vi "I2C_0208.vi"() -> ()   [LabVIEW 2021]
doc: "This example demonstrates how to generate a user-defined voltage using the analog output of a DAQ device."
uses:
  <vilib>/Utility/error.llb/DialogType.ctl
  <vilib>/DAQmx/write.llb/DAQmx Write (Digital 1D U32 1Chan NSamp).vi
  <vilib>/DAQmx/create/channels.llb/DAQmx Create Channel (DO-Digital Output).vi
  <vilib>/DAQmx/configure/timing.llb/DAQmx Timing (Sample Clock).vi
  <vilib>/DAQmx/miscellaneous.llb/DAQmx Fill In Error Info.vi
  <vilib>/Utility/file.llb/Read Delimited Spreadsheet (I64).vi
  <vilib>/DAQmx/write.llb/DAQmx Write (Digital 1D U32 NChan 1Samp).vi
  <resource>/objmgr/daqmx.rc
panel:
  out "Time Pass Outside":u32
  out "Time Pass Inside":u32
  in  "lines":tag
  in  "source":tag
  in  "rate":dbl=1000.0 format="%0.2f"
  out "SampClk.Rate":dbl
  out "DUT":i32
  out "Boolean array":bool[](array[boolean])
  in  "STOP":bool
  out "DIO":cluster{i16, i16}(graph)
  in  "file path (dialog if empty)":path=path "C:/Users/Wayne Shih/Downloads/nPM6100 Positron/HTOL/Labview/AWG by USB6259/test.txt"
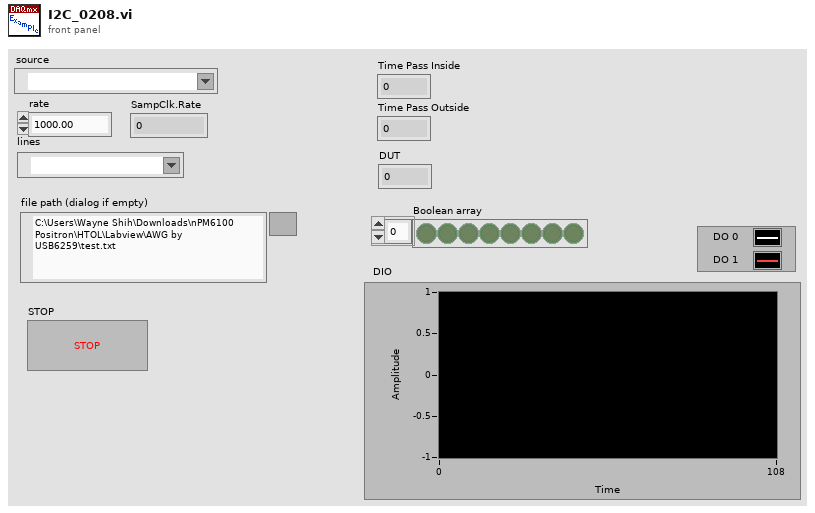
[diagram p1: front panel]
types:
  T1 = typedef "DialogType.ctl" = u16
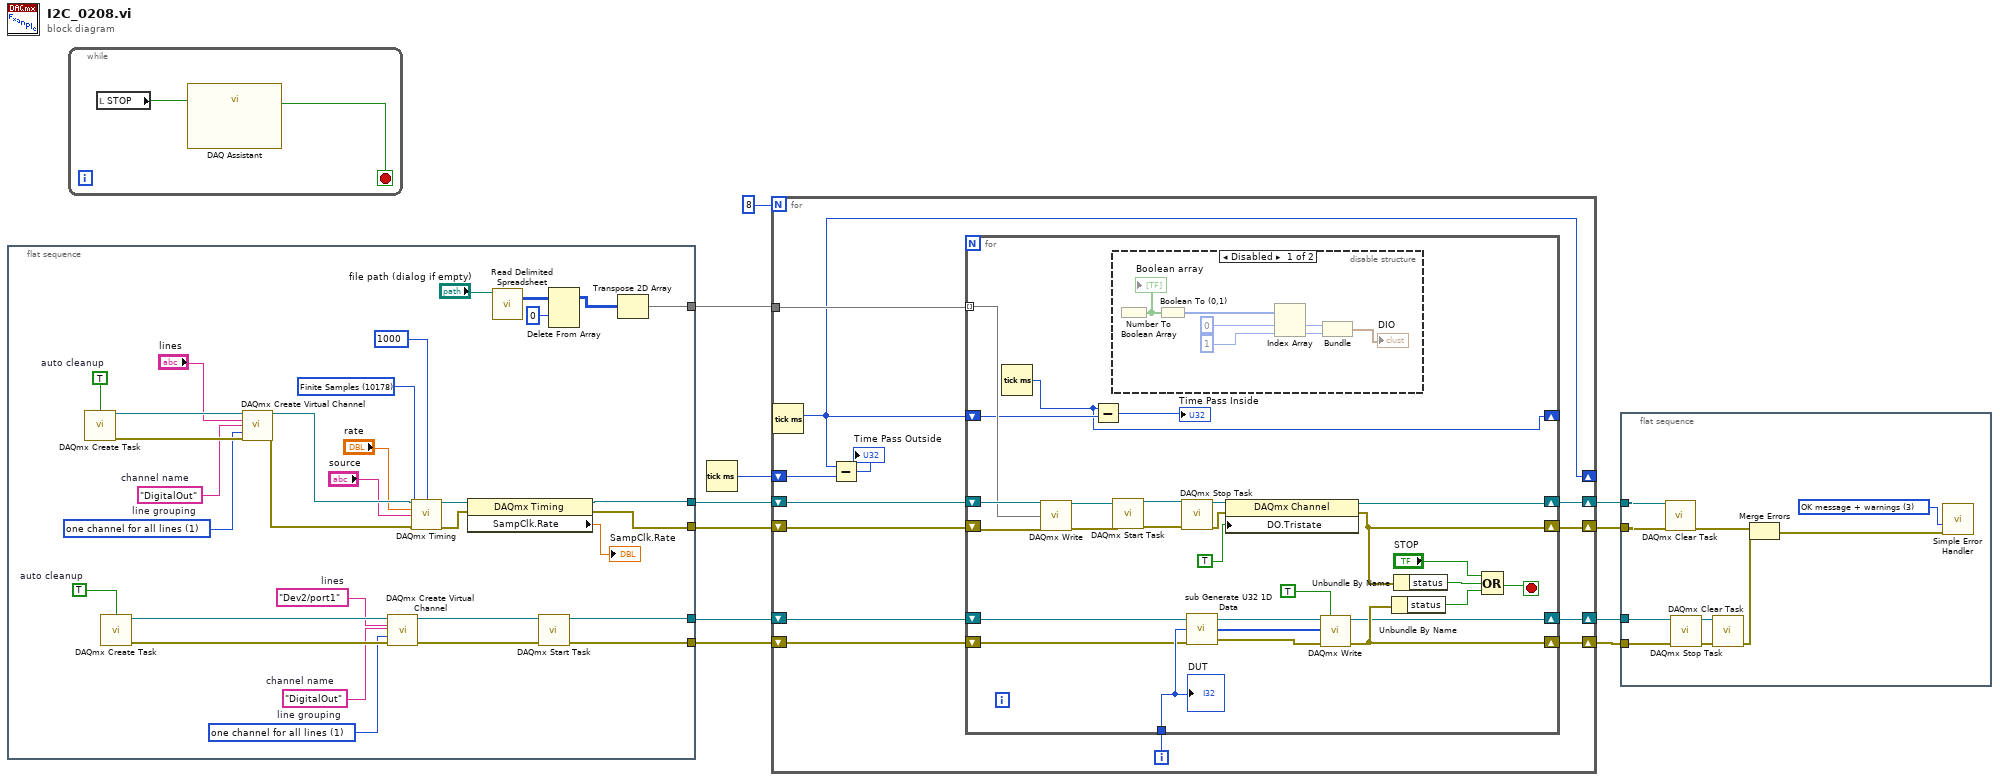
[diagram p0: block diagram]
diagram:
  n1 = flat-sequence {
    tunnel: [w32] -> w11
    tunnel: [w31] -> w10
    tunnel: [w38] -> w8
    tunnel: [w37] -> w7
    tunnel: [w22] -> w2
    frame #0 {
      w15 = 1 items=["one channel for each line", "one channel for all lines"]  # line grouping
      w14 = "DigitalOut"  # channel name
      w16 = "Dev2/port1"  # lines
      w18 = TRUE  # auto cleanup
      w28 = 10178 items=["Finite Samples"=10178, "Continuous Samples"=10123, "Hardware Timed Single Point"=12522] ("sample mode")
      w40 = 1 items=["one channel for each line", "one channel for all lines"]  # line grouping
      w39 = "DigitalOut"  # channel name
      w42 = TRUE  # auto cleanup
      n2 = call <vilib>:"DAQmx Create Task.vi"("auto cleanup"=w42) -> ("task out"=w41:refnum<k21>, "error out"=w43:errorcluster)  [unwired: 13 in]
      n3 = call <vilib>:"DAQmx Create Task.vi"("auto cleanup"=w18) -> ("task out"=w17:refnum<k21>, "error out"=w19:errorcluster)  [unwired: 13 in]
      n4 = call-poly <vilib>:"DAQmx Create Virtual Channel.vi"("task in"=w41, "lines"="lines", "name to assign"=w39, "line grouping"=w40, "error in"=w43) -> ("task out"=w36:refnum<k21>, "error out"=w35:errorcluster)  [unwired: 9 in]
      n5 = call-poly <vilib>:"DAQmx Create Virtual Channel.vi"("task in"=w17, "lines"=w16, "name to assign"=w14, "line grouping"=w15, "error in"=w19) -> ("task out"=w12:refnum<k21>, "error out"=w13:errorcluster)  [unwired: 9 in]
      n6 = call-poly <vilib>:"DAQmx Timing.vi"("task/channels in"=w36, "sample mode"=w28, "samples per channel"=1000, "rate"="rate", "source"="source", "error in"=w35) -> ("task out"=w34:refnum<k21>, "error out"=w33:errorcluster)  [unwired: 8 in]
      n7 = property class="DAQmx Timing"(reference=w34, error in=w33) -> (reference out=w32:refnum<k21>, error out=w31:errorcluster, "SampClk.Rate"=→"SampClk.Rate":dbl)
      n8 = call-poly <vilib>:"Read Delimited Spreadsheet.vi"("file path (dialog if empty)"="file path (dialog if empty)") -> ("all rows"=w25:i64[][])  [unwired: 9 in, 5 out]
      n9 = call <vilib>:"DAQmx Start Task.vi"("task/channels in"=w12, "error in"=w13) -> ("task out"=w38:refnum<k21>, "error out"=w37:errorcluster)  [unwired: 12 in]
      n10 = Delete From Array(array=w25, index (row)=0) -> (array with subset deleted=w24:i64[][])  [unwired: 2 in, 1 out]
      n11 = Transpose 2D Array(2D array=w24) -> (transposed array=w22:i64[][])
    }
  }
  n12 = while {
    stop <- w45 stop-if-true
    n13 = local read "STOP"() -> (w44:bool)
    n14 = call "DAQ Assistant"("stop (F)"=w44) -> ("stopped"=w45:bool)  [unwired: 16 in, 2 out]
  }
  n15 = Tick Count (ms)() -> (millisecond timer value=w1:u32)
  n16 = for {
    N: 8 -> [_]
    shift-right: [w56] -> w4
    shift-left: w11 -> [w58]
    shift-right: [w55] -> w3
    shift-left: w10 -> [w57]
    shift-right: [w51] -> w5
    shift-left: w8 -> [w50]
    shift-right: [w52] -> w6
    shift-left: w7 -> [w53]
    tunnel: w2 -> [w49]
    shift-right: [w47] -> _
    shift-left: w1 -> [w48]
    i -> [w54]
    n17 = Tick Count (ms)() -> (millisecond timer value=w47:u32)
    n18 = Subtract(x=w47, y=w48) -> (x-y=→"Time Pass Outside":u32)
    n19 = for {
      tunnel: w49 -> [w70] mode=indexing
      shift-right: [w60] -> w56
      shift-left: w58 -> [w73]
      shift-right: [w59] -> w55
      shift-left: w57 -> [w72]
      tunnel: w54 -> [w85]
      shift-right: [w82] -> w51
      shift-left: w50 -> [w81]
      shift-right: [w83] -> w52
      shift-left: w53 -> [w84]
      shift-right: [w66] -> _
      shift-left: w47 -> [w68]
      stop <- w71 stop-if-true
      n20 = Tick Count (ms)() -> (millisecond timer value=w66:u32)
      n21 = call-poly <vilib>:"DAQmx Write.vi"("task/channels in"=w73, "data"=w70, "error in"=w72) -> ("task out"=w86:refnum<k21>, "error out"=w69:errorcluster)  [unwired: 10 in, 1 out]
      n22 = Subtract(x=w66, y=w68) -> (x-y=→"Time Pass Inside":u32)
      n23 = disable-structure shown="Disabled" {
        frame Disabled {
          n24 = Number To Boolean Array() -> (Boolean array=w87:bool[])  [unwired: 1 in]
          "Boolean array" <- w87
          n25 = Boolean To (0,1)(Boolean=w87) -> (0, 1=w93:i16[])
          n26 = Index Array(array=w93, index #1=0 ("index"), index #2=1 ("index")) -> (element #1=w90:i16, element #2=w89:i16)
          n27 = Bundle(w90, w89) -> (→"DIO":cluster{i16, i16})  [unwired: 1 in]
        }
        frame Enabled {
        }
      }
      n28 = call <vilib>:"DAQmx Start Task.vi"("task/channels in"=w86, "error in"=w69) -> ("task out"=w64:refnum<k21>, "error out"=w63:errorcluster)  [unwired: 12 in]
      n29 = call <vilib>:"DAQmx Stop Task.vi"("task/channels in"=w64, "error in"=w63) -> ("task out"=w62:refnum<k21>, "error out"=w61:errorcluster)  [unwired: 12 in]
      n30 = call <vilib>:"sub Generate U32 1D Data.vi"("error in"=w84, "initial value"=w85, "task in"=w81) -> ("error out"=w78:errorcluster, "Data"=w77:u32[], "task out"=w76:refnum<k21>)
      n31 = property class="DAQmx Channel"(reference=w62, error in=w61, "DO.Tristate"=TRUE) -> (reference out=w60:refnum<k21>, error out=w59:errorcluster)
      n32 = call-poly <vilib>:"DAQmx Write.vi"("task/channels in"=w76, "auto start"=TRUE, "data"=w77, "error in"=w78) -> ("task out"=w82:refnum<k21>, "error out"=w83:errorcluster)  [unwired: 9 in, 1 out]
      n33 = Unbundle By Name(w83) -> ("status"=w75:bool)
      n34 = Unbundle By Name(w59) -> ("status"=w79:bool)
      n35 = Compound Arithmetic op=OR("STOP", w79, w75) -> (w71:bool)
      "DUT" <- w85
    }
  }
  n36 = flat-sequence {
    tunnel: w4 -> [w95]
    tunnel: w3 -> [w96]
    tunnel: w6 -> [w100]
    tunnel: w5 -> [w99]
    frame #0 {
      w103 = T1 3 items=["no dialog", "OK message", "continue or stop message", "OK message + warnings", "continue/stop + warnings"] ("type of dialog (OK msg:1)")
      n37 = call <vilib>:"DAQmx Clear Task.vi"("task in"=w95, "error in"=w96) -> ("error out"=w97:errorcluster)  [unwired: 13 in]
      n38 = call <vilib>:"DAQmx Stop Task.vi"("task/channels in"=w99, "error in"=w100) -> ("task out"=w101:refnum<k21>, "error out"=w102:errorcluster)  [unwired: 12 in]
      n39 = call <vilib>:"DAQmx Clear Task.vi"("task in"=w101, "error in"=w102) -> ("error out"=w98:errorcluster)  [unwired: 13 in]
      n40 = Merge Errors(w97, w98) -> (w94:errorcluster)
      n41 = call <vilib>:"Simple Error Handler.vi"("type of dialog (OK msg:1)"=w103, "error in (no error)"=w94) -> ()  [unwired: 3 in, 5 out]
    }
  }
